vi "禹山浊度_获取温度和测量值.vi"(8 "error in (no error)":errorcluster caption="错误输入（无错误）", 11 "MB session in":refnum<class "MB_Master.lvclass">) -> (0 "error out":errorcluster caption="错误输出", 2 "输出值":cluster{"温度测量值":sgl, "浊度":sgl}, 3 "MB session out":refnum<class "MB_Master.lvclass">)   [LabVIEW 2016, in "斯坦道多参数.lvlib"]
uses:
  <vilib>/Plasmionique/MB Master/MB_Master/MB_Master.lvclass
  <vilib>/Plasmionique/MB Master/MB Master.lvlib
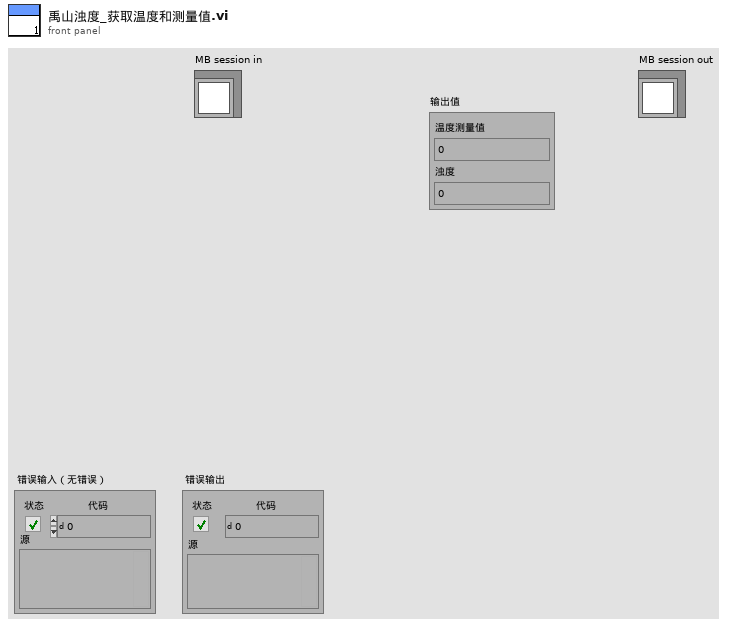
[diagram p1: front panel]
types:
  T1 = cluster{"pH":u32, "DO":u32, "Cond":u32, "Turb":u32, "叶绿素a":u32, "藻密度":u32, "ORP":u32, "COD":u32}
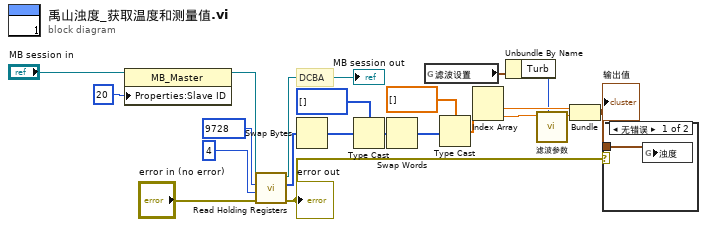
[diagram p0: block diagram]
diagram:
  # "DCBA"
  n1 = property class="MB_Master"(reference="MB session in", "Properties:Slave ID"=u16 20 ("y")) -> (reference out=w13:refnum<class "MB_Master.lvclass">)  [unwired: 1 in, 1 out]
  n2 = call <vilib>:"Read Holding Registers.vi"("error in (no error)"="error in (no error)", "quantity"=u16 4, "starting address"=u16 9728, "MB session in"=w13) -> ("error out"=w8:errorcluster, "Registers"=w11:u16[], "MB session out"=→"MB session out":refnum<class "MB_Master.lvclass">)  [unwired: 5 in]
  "error out" <- w8
  n3 = Swap Bytes(anything=w11) -> (byte swapped=w10:u16[])
  n4 = Type Cast(type=u32[] [] ("数组 2"), x=w10) -> (*(type *) &x=w17:u32[])
  n5 = Swap Words(1:w17) -> (0:w19:u32[])
  n6 = global read "断电保存变量.vi" "滤波设置"() -> (w2:T1)
  n7 = Type Cast(type=sgl[] [] ("数组 2"), x=w19) -> (*(type *) &x=w15:sgl[])
  n8 = Index Array(array=w15) -> (element #1=w9:sgl, element #2=w4:sgl)  [unwired: 2 in]
  n9 = Unbundle By Name(w2) -> ("Turb"=w1:u32)
  n10 = call "滤波参数.vi"("滤波次数"=w1, "x"=w4) -> ("mode"=w3:dbl)  [unwired: 9 in]
  n11 = Bundle("数值"=w9, "mode"=w3) -> (w7:cluster{"数值":sgl, "mode":dbl})  [unwired: 1 in]
  "输出值" <- w7
  n12 = case shown="无错误" w8 {
    tunnel: w7 -> [w22 _]
    frame No Error {
      n13 = global write "禹山过程全局变量.vi" "浊度"(w22) -> ()
    }
    frame Error {
    }
  }
